vi "PCO_GetShutterMode.vi"(8 "error in (no error)":errorcluster {"code" format="%x"}, 11 "ph":u64) -> (0 "error out":errorcluster {"code" format="%x"}, 1 "wShutterMode":u16(ring)=1 items=["Rolling Shutter"=1, "Global Shutter"=2, "Global Reset"=4], 2 "ErrorMessage":i32 format="%x", 3 "ph out":u64)   [LabVIEW 2019, in "SDK.lvlib" / "GeneralCameraControl.lvlib"]
doc: "<b>Description:</b>\nThis function will reboot the camera. The function will return immediately and the reboot process in the camera is started. After calling this command the handle to this camera should be closed with PCO_CloseCamera.\nWhen reboot is finished (approximately after 6 to 10 seconds, up to 40 seconds for cameras with GigE interface) the camera can be reopened with a PCO_OpenCameraEx call. The reboot command is used during firmware update and is necessary when camera setup is changed.\n\n<b>Supported camera type:</b>\nAll cameras\n\n<b>Descriptor dependency:</b>\nNone"
uses:
  GeneralCameraControl.lvlib
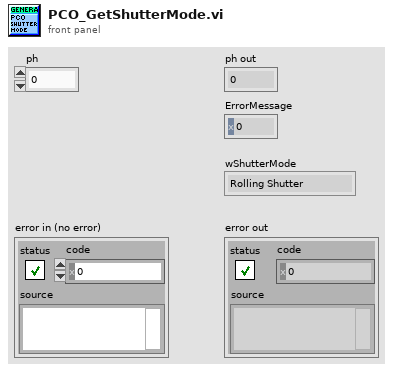
[diagram p1: front panel]
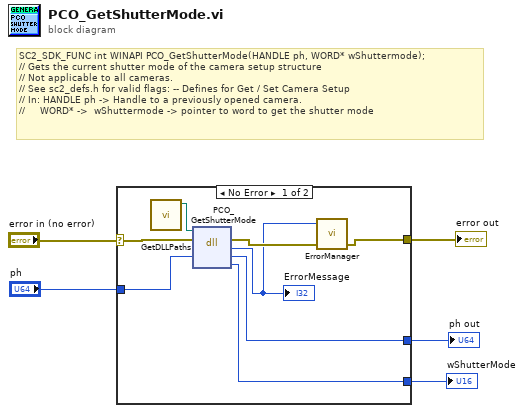
[diagram p0: block diagram]
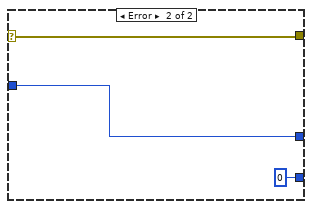
[diagram p2: hidden frame]
diagram:
  # "SC2_SDK_FUNC int WINAPI PCO_GetShutterMode(HANDLE ph, WORD* wShuttermode);\n// Gets the current shutter mode of the camera setup structure\n// Not applicable to all cameras.\n// See sc2_defs.h for valid flags: -- Defines for Get / Set Camera Setup\n// In: HANDLE ph -> Handle to a previously opened camera.\n//     WORD* ->  wShuttermode -> pointer to word to get the shutter mode"
  n1 = case shown="No Error" "error in (no error)" {
    selector: "error in (no error)" -> [w11 w15]
    tunnel: "ph" -> [w13 w16]
    tunnel: [w12 w16] -> w4
    tunnel: [w9 w15] -> w2
    tunnel: [w6 u16 0 ("wShutterMode")] -> w1
    frame No Error {
      n2 = call "GetDLLPaths.vi"() -> ("SC2_Cam_Path"=w7:path)  [unwired: 8 in, 3 out]
      n3 = dll-call lib="?" fn="PCO_GetShutterMode"(path in=w7, error in=w11, "ph"=w13) -> (error out=w10:errorcluster, "return type"=w8:i32, "ph"=w12:u64, "wShutterMode"=w6:u16)  [unwired: 2 in, 1 out]
      "ErrorMessage" <- w8
      n4 = call "ErrorManager.vi"("error in (no error)"=w10, "error code"=w8) -> ("error out"=w9:errorcluster)  [unwired: 2 in, 1 out]
    }
    frame Error {
    }
  }
  "ph out" <- w4
  "error out" <- w2
  "wShutterMode" <- w1
